vi "WPI_CameraGet Sharpness.vi"(8 "error in (no error)":errorcluster, 11 "CameraDevRef":T1={"Camera Address"="192.168.0.90", "CameraStatus"={"status"=FALSE, "code"=0, "source"=""}}) -> (0 "error out":errorcluster, 2 "Sharpness":i32, 3 "CameraDevRef Out":T1)   [LabVIEW 2017]
doc: "Returns the sharpness setting of the camera you specify.\n\nThis software is licensed. Open the labview\\readme\\WPI Robotics Library Open Source License.txt file for more information."
uses:
  <vilib>/Rock Robotics/WPI/Camera/WPI_CameraDevRef.ctl
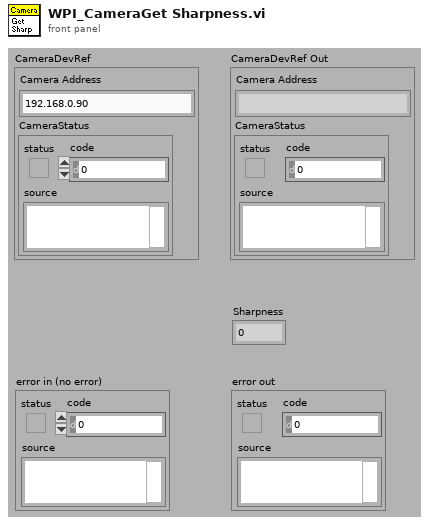
[diagram p1: front panel]
types:
  T1 = typedef "WPI_CameraDevRef.ctl" = cluster{"Camera Address":string, "CameraStatus":errorcluster}
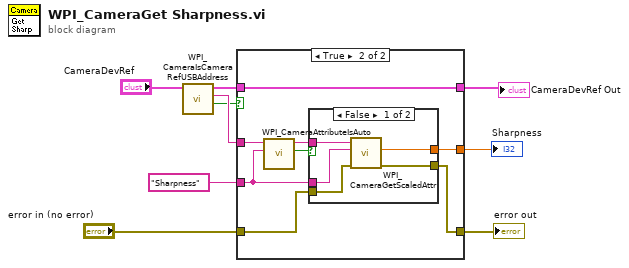
[diagram p0: block diagram]
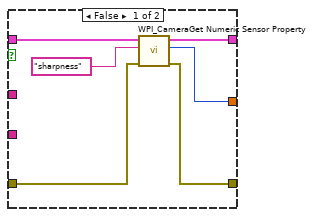
[diagram p2: hidden frame]
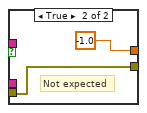
[diagram p3: hidden frame]
diagram:
  n1 = call <vilib>:"WPI_CameraIsCameraRefUSBAddress.vi"("CameraDevRef"="CameraDevRef") -> ("USB?"=w1:bool, "Camera Address Out"=w2:string, "CameraDevRef out"=w3:T1)  [unwired: 7 in, 1 out]
  n2 = case shown="True" w1 {
    tunnel: w3 -> [w15 w23]
    tunnel: [w14 w23] -> w9
    tunnel: [w13 w18] -> w8
    tunnel: "error in (no error)" -> [w12 w17]
    tunnel: [w11 w16] -> w6
    tunnel: w2 -> [_ w22]
    tunnel: "Sharpness" -> [_ w20]
    frame False {
      n3 = call <vilib>:"WPI_CameraGet Numeric Sensor Property.vi"("error in (no error)"=w12, "Property Name"="sharpness", "CameraDevRef"=w15) -> ("error out"=w11:errorcluster, "Value"=w13:i32, "CameraDevRef dup"=w14:T1)  [unwired: 2 in, 4 out]
    }
    frame True {
      n4 = call <vilib>:"WPI_CameraAttributeIsAuto.vi"("Attr String"=w20, "Camera Address In"=w22) -> ("Auto?"=w21:bool, "Camera Address Out"=w19:string)  [unwired: 8 in]
      n5 = case shown="False" w21 {
        tunnel: w20 -> [w27 _]
        tunnel: w19 -> [w28 _]
        tunnel: [w26 -1.0] -> w18
        tunnel: w17 -> [w25 w29]
        tunnel: [w24 w29] -> w16
        frame False {
          n6 = call <vilib>:"WPI_CameraGetScaledAttr.vi"("error in (no error)"=w25, "Attr String"=w27, "Camera Address In"=w28) -> ("error out"=w24:errorcluster, "Scaled"=w26:dbl)  [unwired: 5 in, 2 out]
        }
        frame True {
          # "Not expected"
        }
      }
    }
  }
  "CameraDevRef Out" <- w9
  "Sharpness" <- w8
  "error out" <- w6
